vi "Get Screen Bounds.vi"() -> (2 "Height":i32, 3 "Width":i32)   [LabVIEW 2021]
uses:
  System.Windows.Forms
  System.Drawing
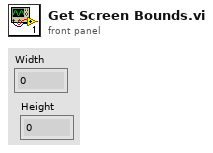
[diagram p1: front panel]
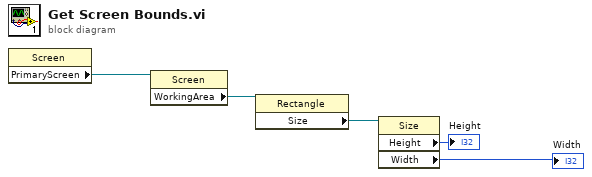
[diagram p0: block diagram]
diagram:
  n1 = property class="Screen"() -> ("PrimaryScreen"=w5:refnum<k24>)  [unwired: 2 in, 2 out]
  n2 = property class="Screen"(reference=w5) -> ("WorkingArea"=w4:refnum<k24>)  [unwired: 1 in, 2 out]
  n3 = property class="Rectangle"(reference=w4) -> ("Size"=w3:refnum<k24>)  [unwired: 1 in, 2 out]
  n4 = property class="Size"(reference=w3) -> ("Height"=→"Height":i32, "Width"=→"Width":i32)  [unwired: 1 in, 2 out]
